vi "ReadWrite LoopStats.vi"(6 "Iteration Duration":i64, 7 "Mode":T1, 8 "error in (no error)":errorcluster, 11 "RT Data in":T2 {"Label Transfer Config"."Block Data Refs"."Data Reference" format="%.0x"; "Status Config"."HWOut Dur Ref" format="%.0x"; "Status Config"."HWIn Dur Ref" format="%.0x"; "Status Config"."Error Data Ref" format="%.0x"; "HWOutput Channels"."Labels Settings"."Label" format="%.0o"; "HWInput Channels"."Labels Settings"."Label" format="%.0o"}) -> (0 "error out":errorcluster, 3 "RT Data out":T2 {"Label Transfer Config"."Block Data Refs"."Data Reference" format="%.0x"; "Status Config"."HWOut Dur Ref" format="%.0x"; "Status Config"."HWIn Dur Ref" format="%.0x"; "Status Config"."Error Data Ref" format="%.0x"; "HWOutput Channels"."Labels Settings"."Label" format="%.0o"; "HWInput Channels"."Labels Settings"."Label" format="%.0o"})   [LabVIEW 2015, in "AIT 429 Engine.lvlib"]
uses:
  AIT 429 Engine.lvlib
  RT Controls/RT Data.ctl
  RT Controls/RT HW Channel.ctl
  RT Controls/RT Label Settings.ctl
  Shared/Controls and Global/Label.ctl
  Shared/Controls and Global/transferPeriod.ctl
  RT Controls/Driver Data.ctl
  RT Controls/RT Word Settings.ctl
  <vilib>/NI Veristand/Custom Device API/Block Data Reference.ctl
  <vilib>/NI Veristand/Custom Device API/Data Reference.ctl
  RT Controls/RT Param Setting.ctl
  Shared/Controls and Global/Start Bit.ctl
  Shared/Controls and Global/Number of Bits.ctl
  Shared/Controls and Global/TransferType.ctl
  RT Controls/Error Qs.ctl
  RT Controls/Status Channels Config.ctl
  RT Controls/FIFO.ctl
  RT Controls/Label Transfer Config.ctl
  RT Controls/ReadWrite Selector.ctl
  <vilib>/NI Veristand/Custom Device API/Global Data Refs.vi
  <vilib>/NI Veristand/Custom Device API/Custom Device API.lvlib
  Shared/AIT 429 Shared.lvlib
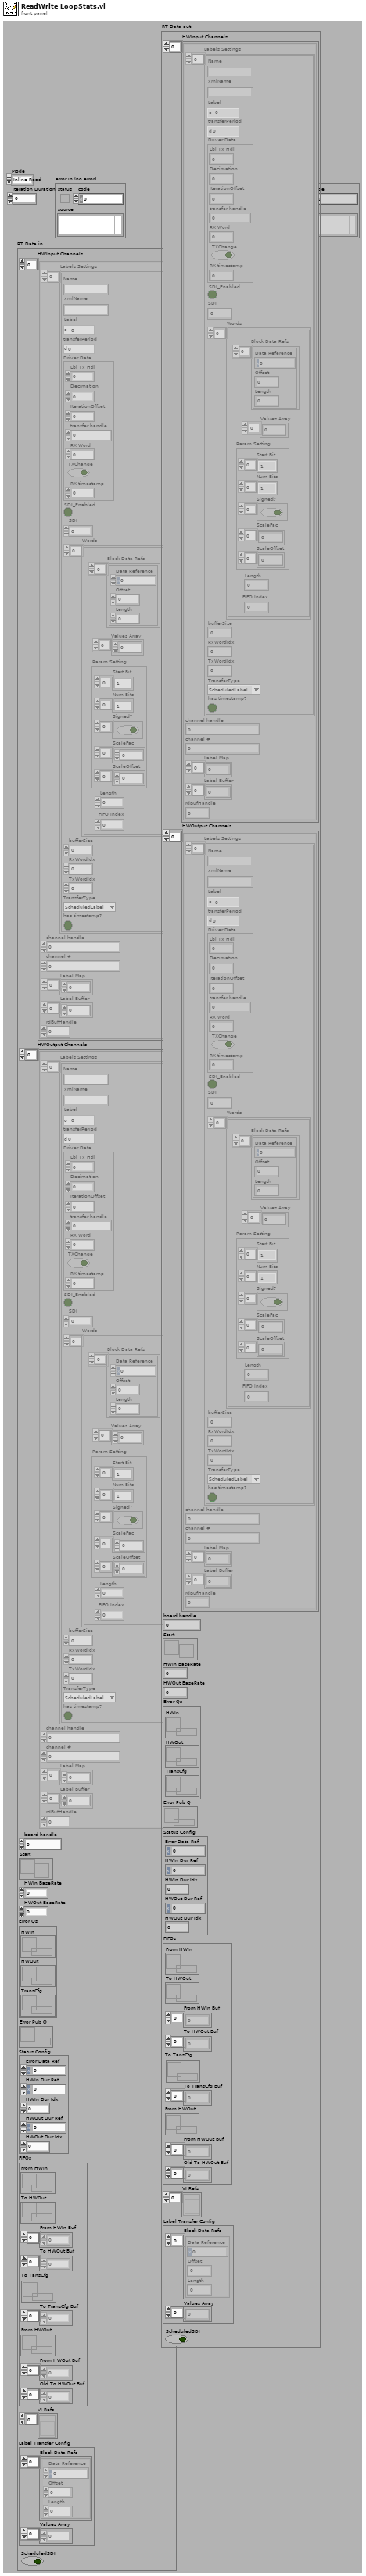
[diagram p1: front panel]
types:
  T1 = typedef "AIT 429 Engine.lvlib/ReadWrite Selector.ctl" = enum16{"Inline Read", "Inline Write", "Async HWIn", "Async HWOut"}
  T2 = typedef "AIT 429 Engine.lvlib/RT Data.ctl" = cluster{"HWInput Channels":T3[], "HWOutput Channels":T3[], "board handle":u32, "Start":refnum<notifier>, "HWIn BaseRate":i64, "HWOut BaseRate":i64, "Error Qs":T15, "Error Pub Q":refnum<queue>, "Status Config":T16, "FIFOs":T17, "VI Refs":refnum<vi>[], "Label Transfer Config":T18, "ScheduledSDI":bool}
  T3 = typedef "AIT 429 Engine.lvlib/RT HW Channel.ctl" = cluster{"Labels Settings":T4[], "channel handle":u32, "channel #":u16, "Label Map":i32[], "Label Buffer":u32[], "rdBufHandle":u32}
  T4 = typedef "AIT 429 Engine.lvlib/RT Label Settings.ctl" = cluster{"Name":string, "xmlName":string, "Label":T5, "transferPeriod":T6, "Driver Data":T7, "SDI_Enabled":bool, "SDI":u8, "Words":T8[], "bufferSize":u32, "RxWordIdx":i32, "TxWordIdx":i32, "TransferType":T14, "has timestamp?":bool}
  T5 = typedef "AIT 429 Shared.lvlib/Label.ctl" = u8
  T6 = typedef "AIT 429 Shared.lvlib/transferPeriod.ctl" = u32
  T7 = typedef "AIT 429 Engine.lvlib/Driver Data.ctl" = cluster{"Lbl Tx Hdl":u32, "Decimation":i32, "IterationOffset":i32, "transfer handle":u32, "RX Word":u32, "TXChange":bool, "RX timestamp":dbl}
  T8 = typedef "AIT 429 Engine.lvlib/RT Word Settings.ctl" = cluster{"Block Data Refs":T9[], "Values Array":dbl[], "Length":i32, "FIFO Index":i32, "Param Setting":T11}
  T9 = typedef "Custom Device API.lvlib/Block Data Reference.ctl" = cluster{"Data Reference":T10, "Offset":u64, "Length":u64}
  T10 = typedef "Custom Device API.lvlib/Data Reference.ctl" = i32
  T11 = typedef "AIT 429 Engine.lvlib/RT Param Setting.ctl" = cluster{"Start Bit":T12[], "Num Bits":T13[], "Signed?":bool[], "ScaleFac":dbl[], "ScaleOffset":dbl[]}
  T12 = typedef "AIT 429 Shared.lvlib/Start Bit.ctl" = i32
  T13 = typedef "AIT 429 Shared.lvlib/Number of Bits.ctl" = i32
  T14 = typedef "AIT 429 Shared.lvlib/TransferType.ctl" = enum16{"ScheduledLabel", "Acyclic", "Block", "Strobe"}
  T15 = typedef "AIT 429 Engine.lvlib/Error Qs.ctl" = cluster{"HWIn":refnum<queue>, "HWOut":refnum<queue>, "TransCfg":refnum<queue>}
  T16 = typedef "AIT 429 Engine.lvlib/Status Channels Config.ctl" = cluster{"Error Data Ref":T10, "HWIn Dur Ref":T10, "HWIn Dur Idx":i32, "HWOut Dur Ref":T10, "HWOut Dur Idx":i32}
  T17 = typedef "AIT 429 Engine.lvlib/FIFO.ctl" = cluster{"From HWIn":refnum<k33>, "To HWOut":refnum<k33>, "From HWIn Buf":dbl[], "To HWOut Buf":dbl[], "To TansCfg":refnum<k33>, "To TransCfg Buf":dbl[], "From HWOut":refnum<k33>, "From HWOut Buf":dbl[], "Old To HWOut Buf":dbl[]}
  T18 = typedef "AIT 429 Engine.lvlib/Label Transfer Config.ctl" = cluster{"Block Data Refs":T9[], "Values Array":dbl[]}
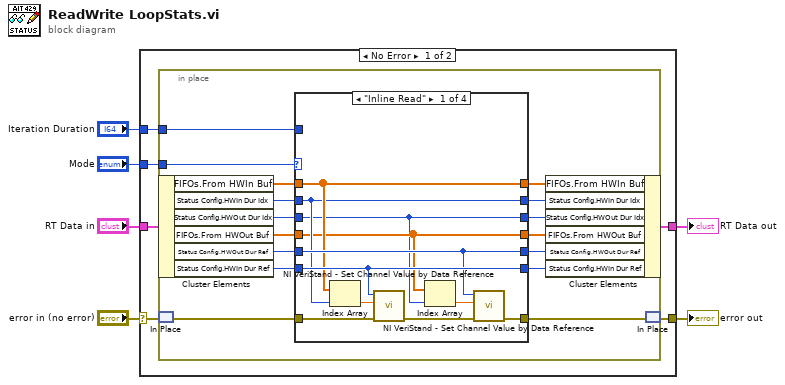
[diagram p0: block diagram]
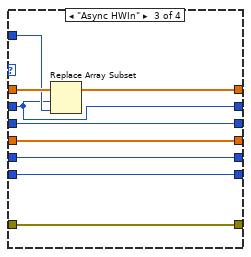
[diagram p3: hidden frame]
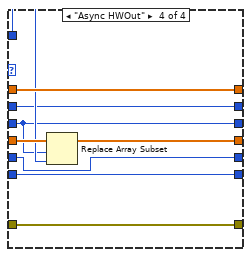
[diagram p4: hidden frame]
diagram:
  n1 = case shown="No Error" "error in (no error)" {
    selector: "error in (no error)" -> [w11 w66]
    tunnel: "RT Data in" -> [w12 w65]
    tunnel: [w10 w65] -> w4
    tunnel: [w9 w66] -> w3
    tunnel: "Mode" -> [w8 _]
    tunnel: "Iteration Duration" -> [w7 _]
    frame No Error {
      n2 = in-place {
        in-place-border: w8 -> [w24]
        in-place-border: w7 -> [w13]
        n3 = in-place-cluster #1(w12) -> ("FIFOs.From HWIn Buf"=w28:dbl[], "Status Config.HWIn Dur Idx"=w21:i32, "Status Config.HWOut Dur Idx"=w18:i32, "FIFOs.From HWOut Buf"=w27:dbl[], "Status Config.HWOut Dur Ref"=w16:T10, "Status Config.HWIn Dur Ref"=w14:T10)
        n4 = in-place-match #2(w11) -> (w26:errorcluster)
        n5 = case shown="\"Inline Read\"" w24 {
          tunnel: w28 -> [w34 w44 w53 w63]
          tunnel: w27 -> [w30 w45 w55 w62]
          tunnel: w26 -> [w39 w46 w54 w64]
          tunnel: [w38 w46 w54 w64] -> w25
          tunnel: [w30 w45 w55 w61] -> w23
          tunnel: [w34 w44 w52 w63] -> w22
          tunnel: w21 -> [w32 w42 w50 w59]
          tunnel: w13 -> [_ _ w51 w60]
          tunnel: [w32 w42 w50 w59] -> w20
          tunnel: [w29 w43 w49 w58] -> w19
          tunnel: w18 -> [w29 w43 w49 w58]
          tunnel: [w35 w41 w48 w57] -> w17
          tunnel: w16 -> [w35 w41 w48 w57]
          tunnel: [w36 w40 w47 w56] -> w15
          tunnel: w14 -> [w36 w40 w47 w56]
          frame "Inline Read" {
            n6 = Index Array(array=w34, index=w32) -> (element=w33:dbl)
            n7 = call <vilib>:"NI VeriStand - Set Channel Value by Data Reference.vi"("error in (no error)"=w39, "Value"=w33, "Data Reference in"=w36) -> ("error out"=w37:errorcluster)  [unwired: 8 in]
            n8 = Index Array(array=w30, index=w29) -> (element=w31:dbl)
            n9 = call <vilib>:"NI VeriStand - Set Channel Value by Data Reference.vi"("error in (no error)"=w37, "Value"=w31, "Data Reference in"=w35) -> ("error out"=w38:errorcluster)  [unwired: 8 in]
          }
          frame Default {
          }
          frame "Async HWIn" {
            n10 = Replace Array Subset(array=w53, new element=w51, index=w50) -> (w52:dbl[])
          }
          frame "Async HWOut" {
            n11 = Replace Array Subset(array=w62, new element=w60, index=w58) -> (w61:dbl[])
          }
        }
        n12 = in-place-cluster #1("FIFOs.From HWIn Buf"=w22, "Status Config.HWIn Dur Idx"=w20, "Status Config.HWOut Dur Idx"=w19, "FIFOs.From HWOut Buf"=w23, "Status Config.HWOut Dur Ref"=w17, "Status Config.HWIn Dur Ref"=w15) -> (w10:T2)
        n13 = in-place-match #2(w25) -> (w9:errorcluster)
      }
    }
    frame Error {
    }
  }
  "error out" <- w3
  "RT Data out" <- w4
